vi "niRFUtil MT UTIL IQ Impairments Validate.vi"(0 "Waveform In":T1={"x0"=0.0, "dx"=1.0, "y"=[]} caption="input complex waveform" {"y" format="%.2f"; "dx" format="%^.2e"; "x0" format="%^.2e"}, 1 "frequency offset (Hz)":dbl, 2 "Quadrature Skew, deg":dbl format="%.2f", 5 "IQ Gain Imbalance, dB":dbl format="%.2f", 7 "Q DC Offset, %":dbl format="%.2f", 9 "I DC Offset, %":dbl format="%.2f") -> (15 "error out":errorcluster)   [LabVIEW 2015, in "niRFUtil.lvlib"]
doc: "This VI validates the inputs for the MT IQ Impairments VI."
uses:
  niRFUtil.lvlib
  Includes/niRFUtil INC Complex Waveform.ctl
  Includes/niRFUtil INC Complex Array.ctl
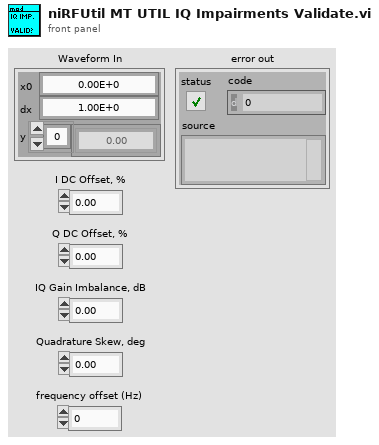
[diagram p1: front panel]
types:
  T1 = typedef "niRFUtil.lvlib/niRFUtil INC Complex Waveform.ctl" = cluster{"x0":dbl, "dx":dbl, "y":T2}
  T2 = typedef "niRFUtil.lvlib/niRFUtil INC Complex Array.ctl" = csg[]
  T3 = cluster{"status":bool, "code":i32, "name":string}[]
  T4 = cluster{"status":bool, "code":i32, "name":string}
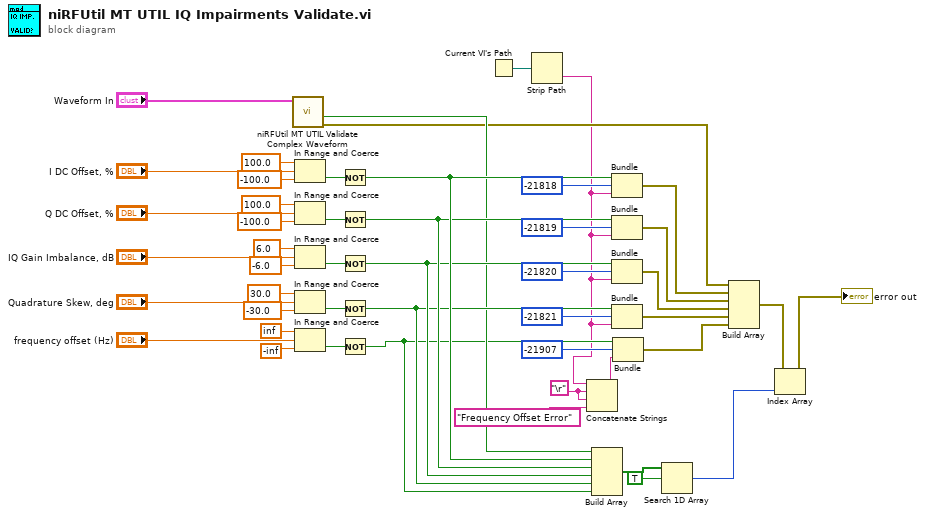
[diagram p0: block diagram]
diagram:
  w1 = "\r"
  n1 = call "niRFUtil MT UTIL Validate Complex Waveform.vi"("Waveform In"="Waveform In") -> ("error out"=w12:errorcluster, "error?"=w13:bool)  [unwired: 1 in, 8 out]
  n2 = In Range and Coerce(upper limit=100.0, x="I DC Offset, %", lower limit=-100.0) -> (In Range?=w46:bool)  [unwired: 1 out]
  n3 = In Range and Coerce(upper limit=100.0, x="Q DC Offset, %", lower limit=-100.0) -> (In Range?=w33:bool)  [unwired: 1 out]
  n4 = In Range and Coerce(upper limit=6.0, x="IQ Gain Imbalance, dB", lower limit=-6.0) -> (In Range?=w26:bool)  [unwired: 1 out]
  n5 = In Range and Coerce(upper limit=30.0, x="Quadrature Skew, deg", lower limit=-30.0) -> (In Range?=w22:bool)  [unwired: 1 out]
  n6 = In Range and Coerce(upper limit=inf, x="frequency offset (Hz)", lower limit=-inf) -> (In Range?=w6:bool)  [unwired: 1 out]
  n7 = Not(x=w46) -> (.not. x?=w35:bool)
  n8 = Not(x=w33) -> (.not. x?=w29:bool)
  n9 = Not(x=w26) -> (.not. x?=w18:bool)
  n10 = Not(x=w22) -> (.not. x?=w17:bool)
  n11 = Not(x=w6) -> (.not. x?=w5:bool)
  n12 = Current VI's Path() -> (path=w45:path)
  n13 = Strip Path(path=w45) -> (name=w3:string)  [unwired: 1 out]
  n14 = Concatenate Strings(w3, w1, w1, "Frequency Offset Error" ("string")) -> (w4:string)
  n15 = Build Array(w13, w35, w29, w18, w17, w5) -> (w42:bool[])
  n16 = Bundle(w35, "code"=-21818, "name"=w3) -> (w40:cluster{bool, "code":i32, "name":string})  [unwired: 1 out]
  n17 = Bundle(w29, "code"=-21819, "name"=w3) -> (w39:cluster{bool, "code":i32, "name":string})  [unwired: 1 out]
  n18 = Bundle(w18, "code"=-21820, "name"=w3) -> (w16:cluster{bool, "code":i32, "name":string})  [unwired: 1 out]
  n19 = Bundle(w17, "code"=-21821, "name"=w3) -> (w15:cluster{bool, "code":i32, "name":string})  [unwired: 1 out]
  n20 = Bundle(w5, "code"=-21907, w4) -> (w10:cluster{bool, "code":i32, string})  [unwired: 1 out]
  n21 = Search 1D Array(1D array=w42, element=TRUE) -> (index of element=w37:i32)  [unwired: 1 out]
  n22 = Build Array(w12, w40, w39, w16, w15, w10) -> (w38:T3)
  n23 = Index Array(array=w38, index=w37) -> (element=→"error out":T4)
